vi "lvgitSettings Dialog.vi"(8 "error in (no error)":errorcluster, 11 "Configuration in":T1={"Hardware Configuration"={"HW Refnum <Replace Me>"="", "Signal Type <Replace Me>"=enum."Sine Wave"}, "Analysis Configuration"={"Statistics"=TRUE}, "New Data Behavior"=enum."Replace"}) -> (0 "error out":errorcluster, 2 "UI Refresh Needed?":bool, 3 "Configuration out":T1={"Hardware Configuration"={"HW Refnum <Replace Me>"="", "Signal Type <Replace Me>"=enum."Sine Wave"}, "Analysis Configuration"={"Statistics"=TRUE}, "New Data Behavior"=enum."Replace"})   [LabVIEW 2012]
doc: "Dialog for selecting user specified settings."
uses:
  controls/lvgitUser Specified Data.ctl
  controls/lvgitHW Configuration.ctl
  controls/lvgitSimulated Signal Type.ctl
  controls/lvgitAnalysis Configuration.ctl
  controls/lvgitNew Data Behavior.ctl
panel:
  in  "Signal Type":u16(ring) items=["Sine Wave", "Square Wave"]
  in  "New Data Behavior":u16(ring) items=["Replace", "Overlay", "Append"]
  in  "Cancel Button":bool
  in  "OK Button":bool
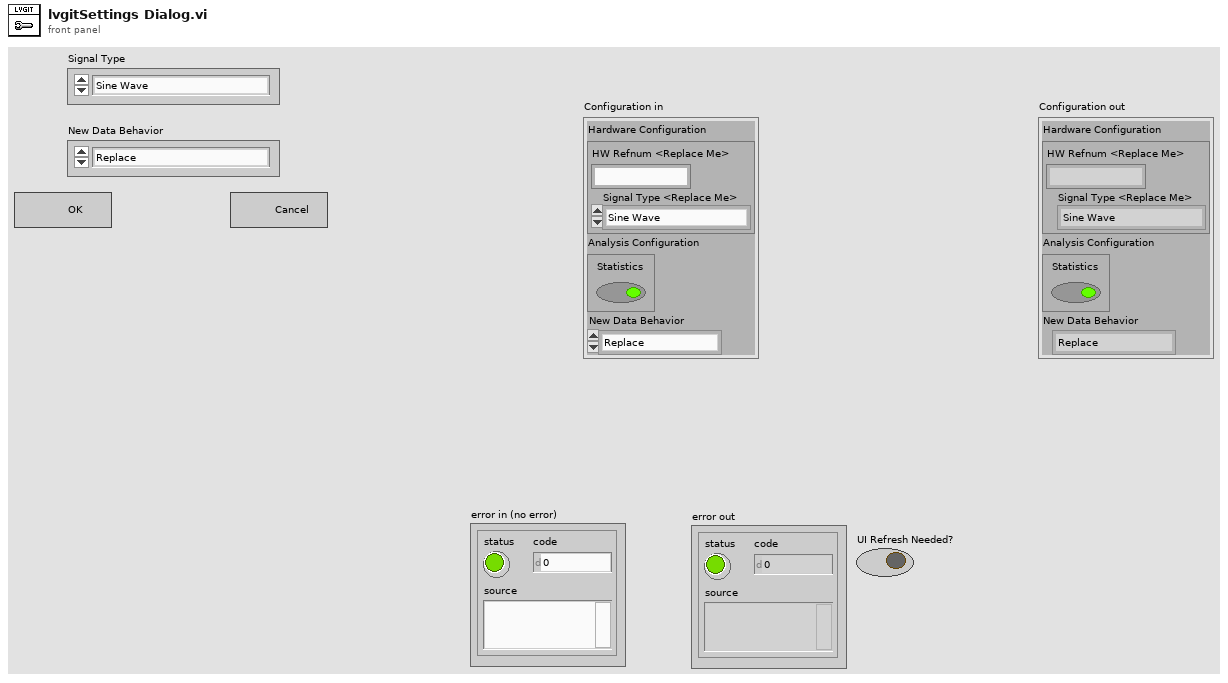
[diagram p1: front panel]
types:
  T1 = typedef "lvgitUser Specified Data.ctl" = cluster{"Hardware Configuration":T2, "Analysis Configuration":T4, "New Data Behavior":T5}
  T2 = typedef "lvgitHW Configuration.ctl" = cluster{"HW Refnum <Replace Me>":string, "Signal Type <Replace Me>":T3}
  T3 = typedef "lvgitSimulated Signal Type.ctl" = enum16{"Sine Wave", "Square Wave"}
  T4 = typedef "lvgitAnalysis Configuration.ctl" = cluster{"Statistics":bool}
  T5 = typedef "lvgitNew Data Behavior.ctl" = enum16{"Replace", "Overlay", "Append"}
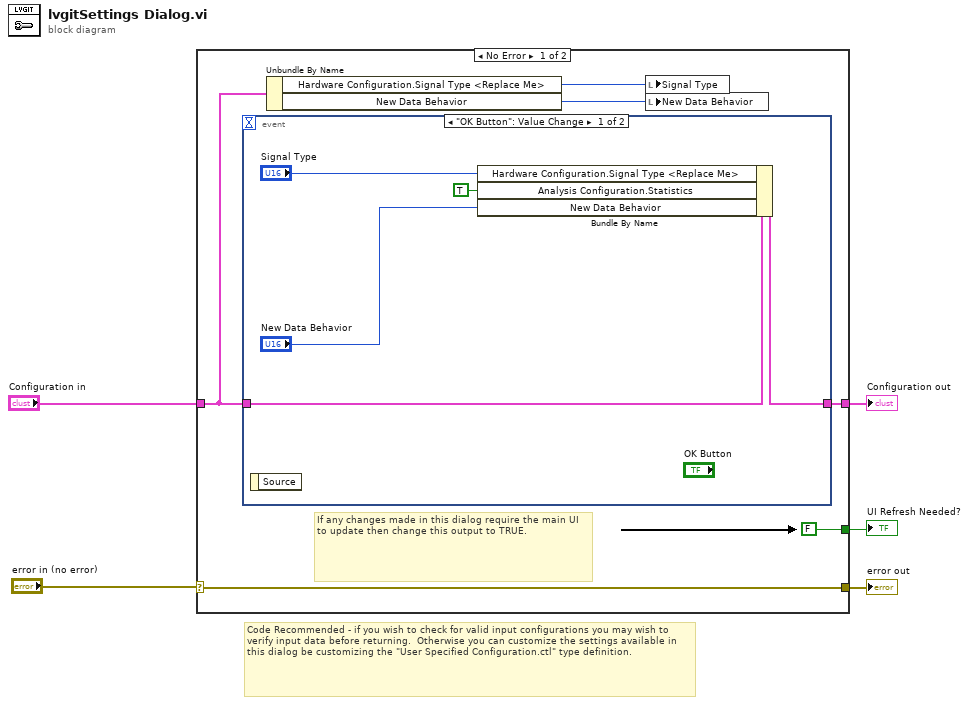
[diagram p0: block diagram]
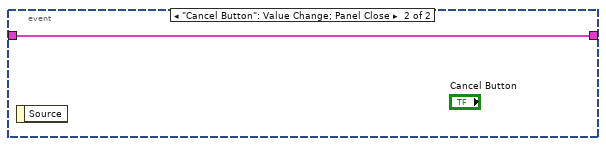
[diagram p2: hidden frame]
diagram:
  # "Code Recommended - if you wish to check for valid input configurations you may wish to verify input data before returning.  Otherwise you can customize the settings available in this dialog be customizing the \"User Specified Configuration.ctl\" type definition."
  n1 = case shown="No Error" "error in (no error)" {
    selector: "error in (no error)" -> [w11 w19]
    tunnel: [w11 w19] -> w4
    tunnel: "Configuration in" -> [w8 w18]
    tunnel: [w10 w18] -> w2
    tunnel: [FALSE ("UI Refresh Needed?") _] -> w1
    frame No Error {
      # "If any changes made in this dialog require the main UI to update then change this output to TRUE."
      n2 = event shown="[0] \"OK Button\": Value Change" {
        selector: _ -> [_ _]
        dyn-events: _ -> [_ _]
        timeout: _ -> [_ _]
        tunnel: [w15 w17] -> w10
        tunnel: w8 -> [w16 w17]
        event "OK Button": Value Change {
          n3 = event-data() -> ()  [unwired: 1 in, 1 out]
          n4 = Bundle By Name(cluster=w16, "Hardware Configuration.Signal Type <Replace Me>"="Signal Type", "Analysis Configuration.Statistics"=TRUE, "New Data Behavior"="New Data Behavior") -> (w15:T1)
        }
        event "Cancel Button": Value Change; Panel Close {
          n5 = event-data() -> ()  [unwired: 1 in, 1 out]
        }
      }
      n6 = Unbundle By Name(w8) -> ("Hardware Configuration.Signal Type <Replace Me>"=w7:T3, "New Data Behavior"=w6:T5)
      n7 = local write "Signal Type"(w7) -> ()
      n8 = local write "New Data Behavior"(w6) -> ()
    }
    frame Error {
    }
  }
  "UI Refresh Needed?" <- w1
  "error out" <- w4
  "Configuration out" <- w2
